vi "Read Element of Channel Names.vi"(8 "error in (no error)":errorcluster, 10 "index":i32, 11 "Temp Control in":refnum<class "Temp Control.lvclass">) -> (0 "error out":errorcluster, 2 "?":string, 3 "Temp Control out":refnum<class "Temp Control.lvclass">)   [LabVIEW 2022 SP3, in "Temp Control.lvclass"]
uses:
  Temp Control.lvclass
  Temp Control.lvclass/Temp Control.ctl
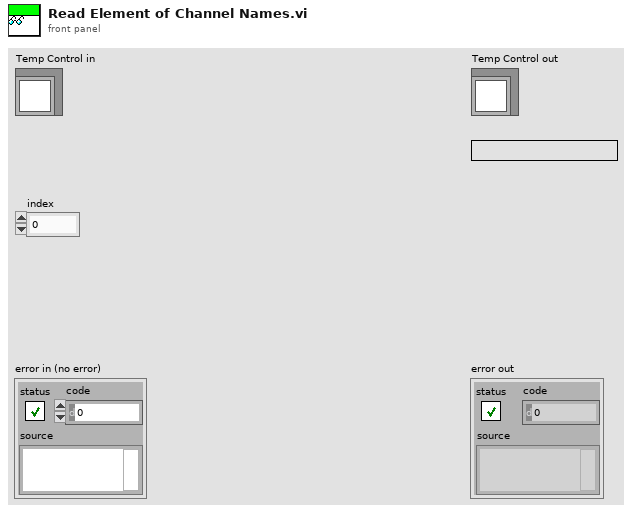
[diagram p1: front panel]
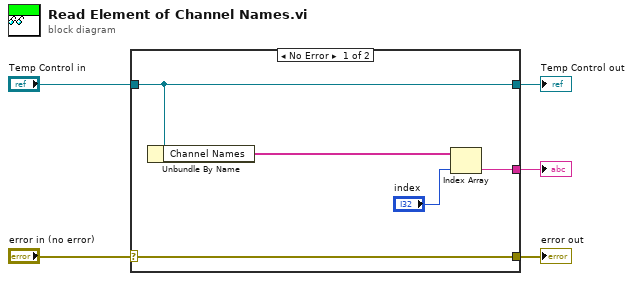
[diagram p0: block diagram]
diagram:
  n1 = case shown="No Error" "error in (no error)" {
    selector: "error in (no error)" -> [w10 w11]
    tunnel: [w10 w11] -> w4
    tunnel: [w9 w12] -> w2
    tunnel: "Temp Control in" -> [w9 w12]
    tunnel: [w6 _] -> w1
    frame No Error {
      n2 = Unbundle By Name(w9) -> ("Channel Names"=w8:string[])
      n3 = Index Array(array=w8, index="index") -> (element=w6:string)
    }
    frame Error {
    }
  }
  "error out" <- w4
  "Temp Control out" <- w2
  "?" <- w1
